vi "AB_Engine_RESTful_Add_Class_Instantiation_VIs.vi"(6 "relative VI paths in":path[](array[path]), 7 "path":path, 8 "error in (no error)":errorcluster, 9 "viConfigs in":T1[](array[typedef]), 10 "destinations":refnum<class "AB_Destination.lvclass">[](array[class]), 11 "buildContext":refnum<vi>) -> (0 "error out":errorcluster, 1 "viConfigs out":T1[](array[typedef]), 4 "relative VI paths out":path[](array[path]))   [LabVIEW 2020]
uses:
  <vilib>/AppBuilder/AB_Classes/Destination/AB_Destination.lvclass
  <vilib>/AppBuilder/AB_Classes/Source/RESTfulVI/Configure_RESTfulVI/AB_RESTful_Configuration.ctl
  <vilib>/AppBuilder/AB_Classes/Source/RESTfulVI/Configure_RESTfulVI/AB_RESTful_VIType.ctl
  <vilib>/AppBuilder/AB_Classes/Source/RESTfulVI/Configure_RESTfulVI/AB_RESTful_OutputType.ctl
  <vilib>/AppBuilder/AB_Classes/Source/RESTfulVI/Configure_RESTfulVI/AB_RESTful_OutputFormat.ctl
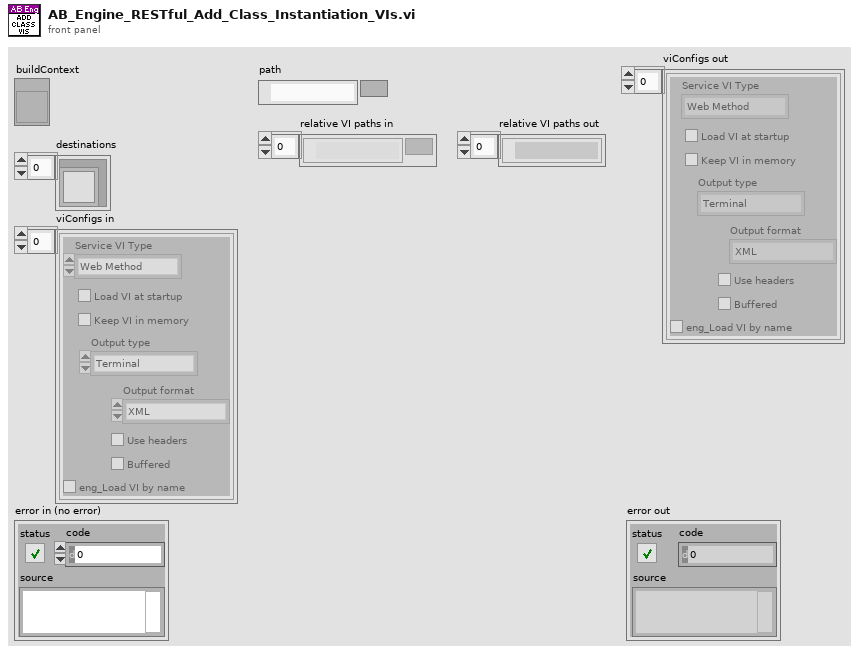
[diagram p1: front panel]
types:
  T1 = typedef "AB_RESTful_Configuration.ctl" = cluster{"Service VI Type":T2, "Load VI at statup":bool, "Keep VI in memory":bool, "Output type":T3, "Output format":T4, "Use headers":bool, "Buffered":bool, "eng_Load VI by name":bool}
  T2 = typedef "AB_RESTful_VIType.ctl" = enum32{"Web Method", "Auxiliary", "eng_Internal", "eng_Content"}
  T3 = typedef "AB_RESTful_OutputType.ctl" = enum32{"Terminal", "Stream"}
  T4 = typedef "AB_RESTful_OutputFormat.ctl" = enum32{"XML", "Text", "HTML", "JSON"}
  T5 = typedef "AB_Destination.ctl" = cluster{"destName":string, "path":path, "libraryName":string, "preserveHierarchy":bool, "eng_inBuild":bool, "eng_libraryReference":refnum<vi>, "eng_restictAddToNewLibrary":bool}
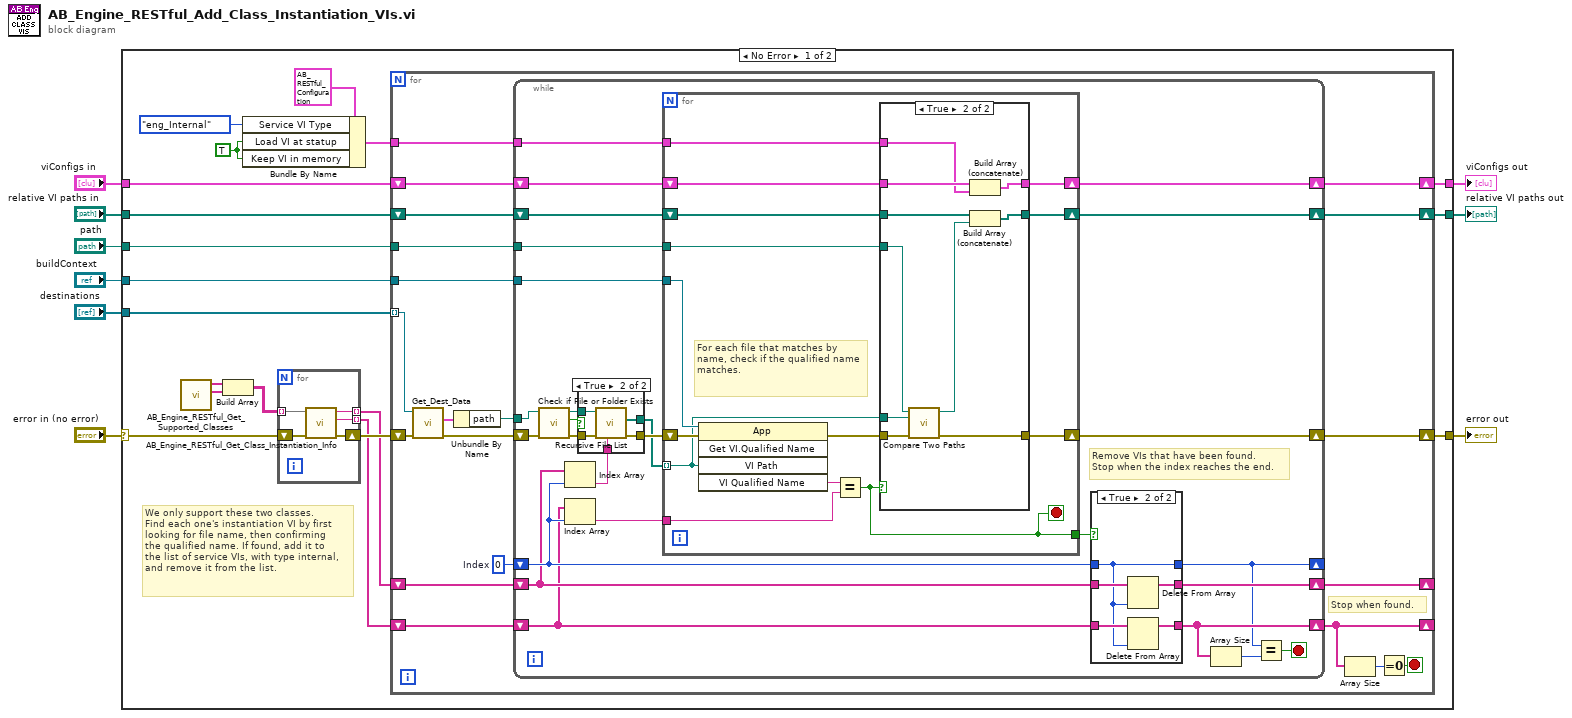
[diagram p0: block diagram]
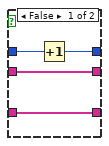
[diagram p3: hidden frame]
diagram:
  n1 = case shown="No Error" "error in (no error)" {
    selector: "error in (no error)" -> [w27 w124]
    tunnel: "destinations" -> [w26 _]
    tunnel: "viConfigs in" -> [w25 w123]
    tunnel: "relative VI paths in" -> [w24 w122]
    tunnel: [w22 w123] -> w5
    tunnel: [w21 w122] -> w4
    tunnel: [w20 w124] -> w3
    tunnel: "buildContext" -> [w19 _]
    tunnel: "path" -> [w16 _]
    frame No Error {
      w15 = TRUE ("Keep VI in memory")
      # "We only support these two classes.\nFind each one's instantiation VI by first\nlooking for file name, then confirming\nthe qualified name. If found, add it to\nthe list of service VIs, with type internal,\nand remove it from the list."
      n2 = call <vilib>:"AB_Engine_RESTful_Get_Supported_Classes.vi"() -> ("Web Request"=w10:string[], "Web Service"=w11:string[])  [unwired: 10 in]
      n3 = Build Array(w11, w10) -> (w28:string[][])
      n4 = Bundle By Name(cluster=T1 {"Service VI Type"=enum."Web Method", "Load VI at statup"=TRUE, "Keep VI in memory"=TRUE, "Output type"=enum."Terminal", "Output format"=enum."XML", "Use headers"=TRUE, "Buffered"=TRUE, "eng_Load VI by name"=FALSE} ("RESTful VI configuration"), "Service VI Type"=AB_RESTful_VIType."eng_Internal", "Load VI at statup"=w15, "Keep VI in memory"=w15) -> (w12:T1)
      n5 = for {
        tunnel: w28 -> [w117] mode=indexing
        shift-right: [w121] -> w23
        shift-left: w27 -> [w120]
        tunnel: [w119] -> w18 mode=indexing
        tunnel: [w118] -> w17 mode=indexing
        n6 = call <vilib>:"AB_Engine_RESTful_Get_Class_Instantiation_Info.vi"("error in (no error)"=w120, "fully qualified LV class name"=w117) -> ("error out"=w121:errorcluster, "qualified instantiation VI name"=w118:string, "instantiation VI file name"=w119:string)  [unwired: 7 in]
      }
      n7 = for {
        tunnel: w26 -> [w48] mode=indexing
        shift-right: [w33] -> w22
        shift-left: w25 -> [w35]
        shift-right: [w32] -> w21
        shift-left: w24 -> [w34]
        shift-right: [w30] -> w20
        shift-left: w23 -> [w47]
        tunnel: w19 -> [w42]
        shift-right: [w41] -> _
        shift-left: w18 -> [w43]
        shift-right: [w36] -> _
        shift-left: w17 -> [w37]
        tunnel: w16 -> [w31]
        tunnel: w12 -> [w29]
        stop <- w39 stop-if-true
        w38 = 0  # Index
        # "Stop when found."
        n8 = call <vilib>:"Get_Dest_Data.vi"("error in (no error)"=w47, "Class in"=w48) -> ("error out"=w44:errorcluster, "destName"=w46:T5)  [unwired: 7 in, 1 out]
        n9 = Unbundle By Name(w46) -> ("path"=w45:path)
        n10 = while {
          tunnel: w45 -> [w51]
          shift-right: [w72] -> w30
          shift-left: w44 -> [w74]
          shift-right: [w59] -> w41
          shift-left: w43 -> [w60]
          tunnel: w42 -> [w71]
          shift-right: [w55] -> _
          shift-left: w38 -> [w68]
          shift-right: [w57] -> w36
          shift-left: w37 -> [w58]
          shift-right: [w64] -> w33
          shift-left: w35 -> [w66]
          shift-right: [w63] -> w32
          shift-left: w34 -> [w65]
          tunnel: w31 -> [w62]
          tunnel: w29 -> [w53]
          stop <- w54 stop-if-true
          # "Remove VIs that have been found.\nStop when the index reaches the end."
          n11 = call <vilib>:"Check if File or Folder Exists.vi"("error in (no error)"=w74, "path"=w51) -> ("error out"=w52:errorcluster, "file or folder exists?"=w49:bool, "dup path"=w50:path)  [unwired: 7 in]
          n12 = Index Array(array=w60, index=w68) -> (element=w69:string)
          n13 = Index Array(array=w58, index=w68) -> (element=w67:string)
          n14 = case shown="True" w49 {
            tunnel: [w75 w80] -> w73
            tunnel: [_ w79] -> w70
            tunnel: w69 -> [_ w78]
            tunnel: w52 -> [w75 w77]
            tunnel: w50 -> [_ w76]
            frame False {
            }
            frame True {
              n15 = call <vilib>:"Recursive File List.vi"("pattern"=w78, "error in (no error)"=w77, "Folder Path"=w76) -> ("error out"=w80:errorcluster, "All Files in Dir"=w79:path[])  [unwired: 4 in, 3 out]
            }
          }
          n16 = for {
            tunnel: w71 -> [w102]
            shift-right: [w98] -> w72
            shift-left: w73 -> [w103]
            tunnel: w70 -> [w92] mode=indexing
            tunnel: w67 -> [w100]
            shift-right: [w96] -> w64
            shift-left: w66 -> [w97]
            shift-right: [w94] -> w63
            shift-left: w65 -> [w95]
            tunnel: w62 -> [w93]
            tunnel: [w91] -> w61
            tunnel: w53 -> [w90]
            stop <- w91 stop-if-true
            # "For each file that matches by name, check if the qualified name matches."
            n17 = invoke class="App" method="Get VI.Qualified Name"(reference=w102, error in=w103, "VI Path"=w92) -> (error out=w99:errorcluster, "VI Qualified Name"=w101:string)  [unwired: 2 in, 3 out]
            n18 = Equal?(x=w101, y=w100) -> (x = y?=w91:bool)
            n19 = case shown="True" w91 {
              tunnel: w99 -> [w104 w116]
              tunnel: [w104 w115] -> w98
              tunnel: w97 -> [w106 w109]
              tunnel: [w106 w108] -> w96
              tunnel: w95 -> [w105 w112]
              tunnel: [w105 w110] -> w94
              tunnel: w93 -> [_ w114]
              tunnel: w92 -> [_ w113]
              tunnel: w90 -> [_ w107]
              frame False {
              }
              frame True {
                n20 = call <vilib>:"Compare Two Paths.vi"("error in (no error)"=w116, "Path 2"=w113, "Path 1"=w114) -> ("error out"=w115:errorcluster, "Relative Path from 1 to 2"=w111:path)  [unwired: 7 out]
                n21 = Build Array (concatenate)(w109, w107) -> (w108:T1[])
                n22 = Build Array (concatenate)(w112, w111) -> (w110:path[])
              }
            }
          }
          n23 = case shown="True" w61 {
            tunnel: [w84 w85] -> w55
            tunnel: w68 -> [w83 w85]
            tunnel: w60 -> [w82 w89]
            tunnel: [w82 w88] -> w59
            tunnel: w58 -> [w81 w87]
            tunnel: [w81 w86] -> w57
            frame False {
              n24 = Increment(x=w83) -> (x+1=w84:i32)
            }
            frame True {
              n25 = Delete From Array(array=w89, index=w85) -> (array with subset deleted=w88:string[])  [unwired: 1 in, 1 out]
              n26 = Delete From Array(array=w87, index=w85) -> (array with subset deleted=w86:string[])  [unwired: 1 in, 1 out]
            }
          }
          n27 = Array Size(array=w57) -> (size(s)=w56:i32)
          n28 = Equal?(x=w55, y=w56) -> (x = y?=w54:bool)
        }
        n29 = Array Size(array=w36) -> (size(s)=w40:i32)
        n30 = Equal To 0?(x=w40) -> (x = 0?=w39:bool)
      }
    }
    frame Error {
    }
  }
  "error out" <- w3
  "relative VI paths out" <- w4
  "viConfigs out" <- w5
